vi "Write Motions Obj.vi"(8 "error in (no error)":errorcluster, 10 "Hardware.lvlib:Motions.lvlib:Motions.lvclass":refnum<class "Motions.lvclass">, 11 "Motions Configuration in":refnum<class "Motions Configuration.lvclass">) -> (0 "error out":errorcluster, 3 "Motions Configuration out":refnum<class "Motions Configuration.lvclass">)   [LabVIEW 2016, in "Hardware.lvlib" / "Motions.lvlib" / "Motions Configuration.lvclass"]
uses:
  <userlib>/Common Components/Hardware/Abstract System/Motions/Motions Config/Motions Configuration.lvclass
  <userlib>/Common Components/Hardware/Abstract System/Motions/Motions/Motions.lvclass
  <userlib>/Common Components/Hardware/Abstract System/Motions/Motions Config/Motions Configuration.lvclass/Motions Configuration.ctl
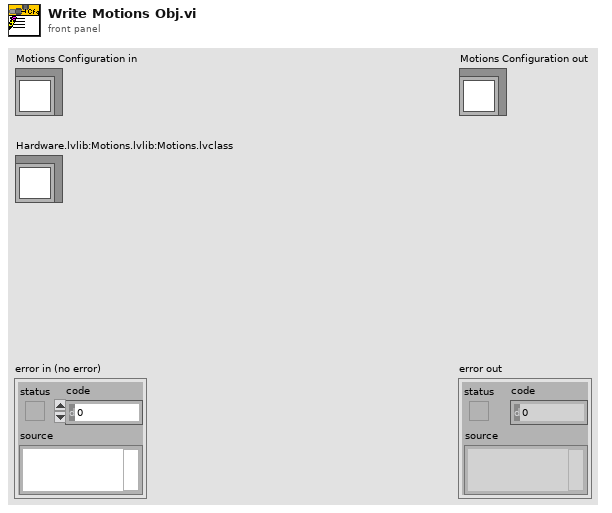
[diagram p1: front panel]
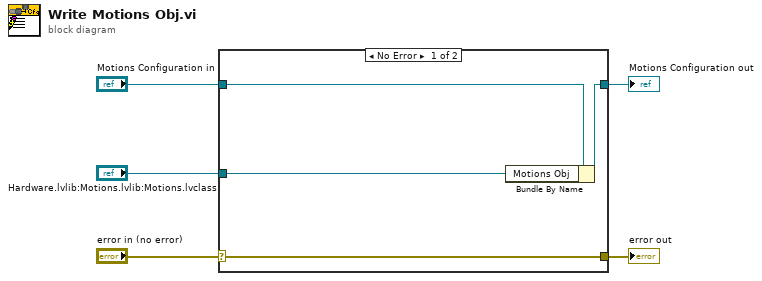
[diagram p0: block diagram]
diagram:
  n1 = case shown="No Error" "error in (no error)" {
    selector: "error in (no error)" -> [w9 w10]
    tunnel: [w9 w10] -> w4
    tunnel: [w7 w11] -> w2
    tunnel: "Motions Configuration in" -> [w8 w11]
    tunnel: "Hardware.lvlib:Motions.lvlib:Motions.lvclass" -> [w6 _]
    frame No Error {
      n2 = Bundle By Name(cluster=w8, "Motions Obj"=w6) -> (w7:refnum<class "Motions Configuration.lvclass">)
    }
    frame Error {
    }
  }
  "error out" <- w4
  "Motions Configuration out" <- w2
